vi "ToWaveformGraph.vi"(8 "error in":errorcluster, 11 "Generic in":refnum<class "Generic.lvclass">) -> (0 "error out":errorcluster, 3 "WFGraph out":refnum<class "WaveformGraph.lvclass">)   [LabVIEW 2014, in "WaveformGraph.lvclass"]
uses:
  WaveformGraph.lvclass
  Generic/Generic.lvclass
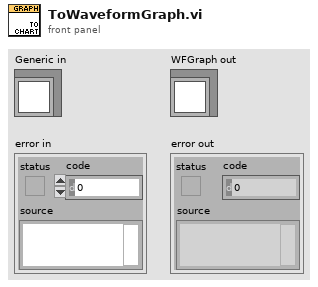
[diagram p1: front panel]
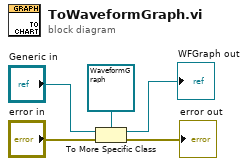
[diagram p0: block diagram]
diagram:
  n1 = To More Specific Class(target class=refnum<class "WaveformGraph.lvclass"> refnum ("RotaryColorScale in 2"), reference="Generic in", error in="error in") -> (specific class reference=→"WFGraph out":refnum<class "WaveformGraph.lvclass">, error out=→"error out":errorcluster)
